vi "testLaserComms_1.vi"() -> ()   [LabVIEW 2015]
panel:
  out "laser power (%)":dbl
  in  "laser power (mW)":dbl
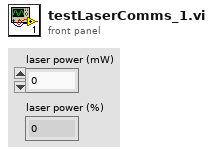
[diagram p1: front panel]
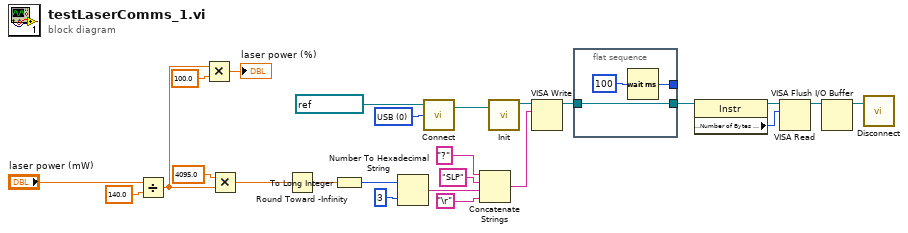
[diagram p0: block diagram]
diagram:
  w24 = u16 0 items=["USB", "RS232"] ("Connection type")
  n1 = Divide(x="laser power (mW)", y=140.0) -> (x/y=w3:dbl)
  n2 = Multiply(x=w3, y=100.0) -> (x*y=→"laser power (%)":dbl)
  n3 = Multiply(x=4095.0 ("number"), y=w3) -> (x*y=w6:dbl)
  n4 = Round Toward -Infinity(1:w6) -> (0:w5:dbl)
  n5 = To Long Integer(number=w5) -> (32bit integer=w4:i32)
  n6 = Number To Hexadecimal String(1:i16 3 ("width (-)"), 2:w4) -> (0:w11:string)
  n7 = call "Connect.vi"("Connection type"=w24, "Com Port"=refnum<visa-resource-name> "COM12") -> ("VISA resource name out"=w25:refnum<visa-resource-name>)  [unwired: 1 in, 1 out]
  n8 = Concatenate Strings("?" ("string"), "SLP" ("Schreibpuffer"), w11, "\r") -> (w19:string)
  n9 = call "Init.vi"("Com Port in"=w25) -> ("COM Port out"=w22:refnum<visa-resource-name>)  [unwired: 1 in, 3 out]
  n10 = VISA Write(VISA resource name=w22, write buffer=w19) -> (VISA resource name out=w18:refnum<visa-resource-name>)  [unwired: 1 in, 2 out]
  n11 = flat-sequence {
    tunnel: w18 -> [w28]
    tunnel: [w28] -> w15
    tunnel: [w26] -> _
    frame #0 {
      n12 = Wait (ms)(milliseconds to wait=u32 100) -> (millisecond timer value=w26:u32)
    }
  }
  n13 = property class="Instr"(reference=w15) -> (reference out=w16:refnum<visa-resource-name>, "Serial Settings:Number of Bytes at Serial Port"=w17:u32)  [unwired: 1 in, 1 out]
  n14 = VISA Read(VISA resource name=w16, byte count=w17) -> (VISA resource name out=w13:refnum<visa-resource-name>)  [unwired: 1 in, 3 out]
  n15 = VISA Flush I/O Buffer(VISA resource name=w13) -> (VISA resource name out=w14:refnum<visa-resource-name>)  [unwired: 2 in, 1 out]
  n16 = call "Disconnect.vi"("Com Port in"=w14) -> ()  [unwired: 1 in, 1 out]
